vi "Problem 17 - Number letter counts.vi"() -> (3 "Answer = no. of letters used for numbers between 1 and 1,000":i32)   [LabVIEW 2021, in "Project Euler.lvlib"]
uses:
  Project Euler.lvlib
  Utilities/Named Timers/Named Timers.lvlib
panel:
  out "Numbers (Proper English)":string[](array[string])
  out "Total execution time (ms)":u32
  # "Development\nControls or indicators that are useful for development or testing, but which are not outputs of the VI."
  # "Input\nInputs to the VI"
  # "Output\nOutputs of the VI"
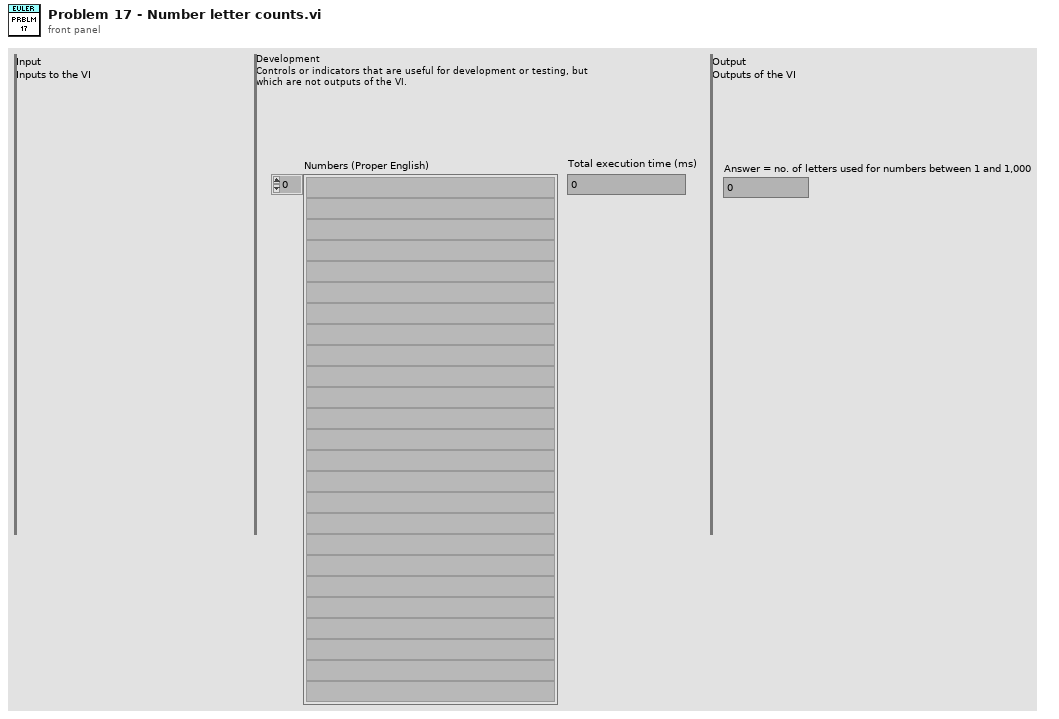
[diagram p1: front panel]
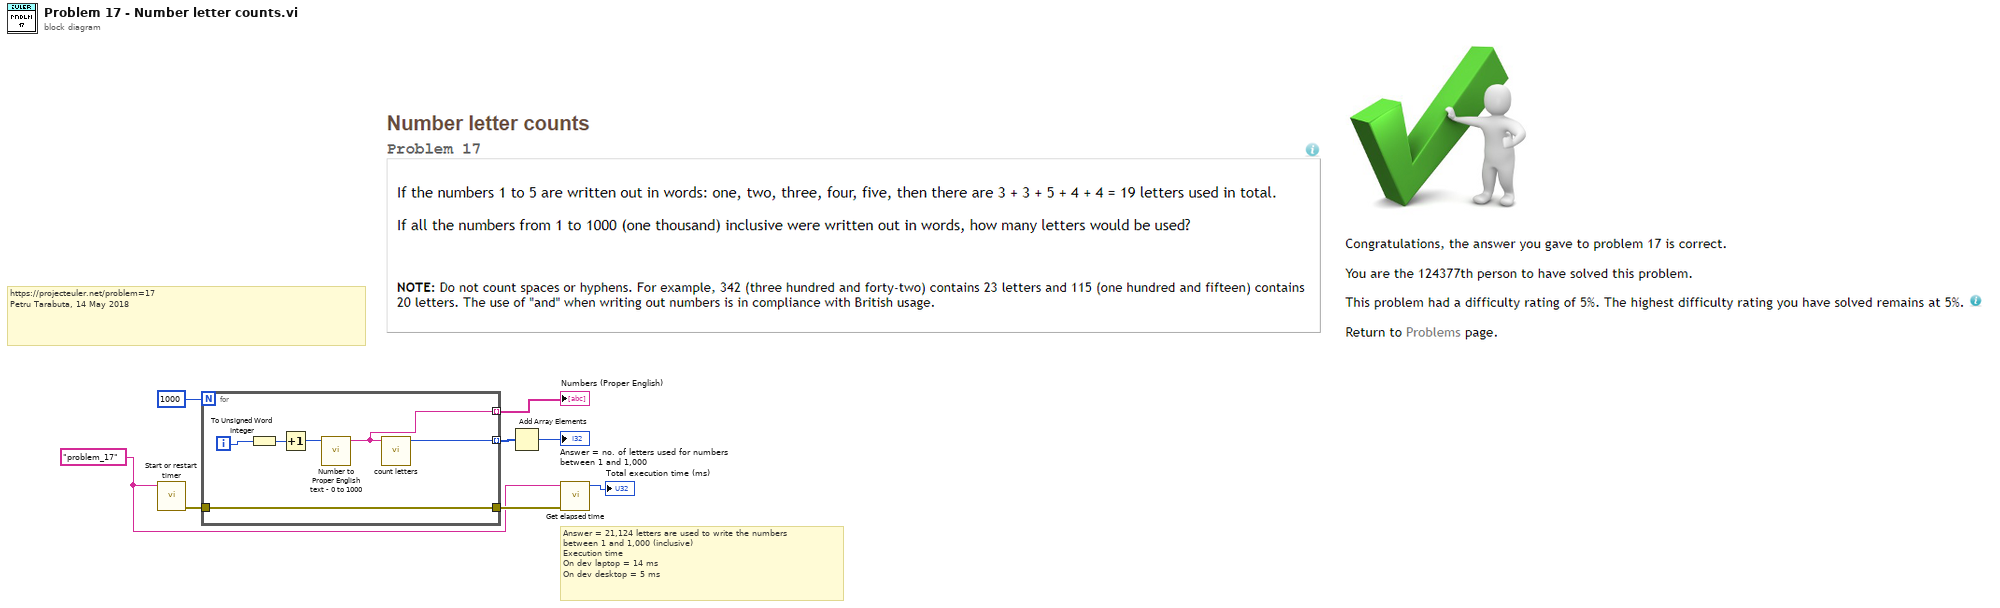
[diagram p0: block diagram]
diagram:
  w1 = "problem_17" ("Timer name")
  # "Answer = 21,124 letters are used to write the numbers between 1 and 1,000 (inclusive)\nExecution time\nOn dev laptop = 14 ms\nOn dev desktop = 5 ms"
  # "https://projecteuler.net/problem=17\nPetru Tarabuta, 14 May 2018"
  n1 = call "Start or restart timer.vi"("Timer name"=w1) -> ("error out"=w3:errorcluster)  [unwired: 10 in]
  n2 = for {
    N: 1000 -> [_]
    tunnel: [w11] -> w6 mode=indexing
    tunnel: [w10] -> w4 mode=indexing
    tunnel: w3 -> [w9]
    tunnel: [w9] -> w2
    i -> [w14]
    n3 = To Unsigned Word Integer(number=w14) -> (unsigned 16bit integer=w12:u16)
    n4 = Increment(x=w12) -> (x+1=w13:u16)
    n5 = call "Number to Proper English text - 0 to 1000.vi"("Positive integer <= 1000"=w13) -> ("Integer written in English"=w11:string)  [unwired: 10 in]
    n6 = call "count letters.vi"("Integer written in English"=w11) -> ("no. of letters"=w10:i32)  [unwired: 10 in]
  }
  "Numbers (Proper English)" <- w6
  n7 = Add Array Elements(numeric array=w4) -> (sum=→"Answer = no. of letters used for numbers between 1 and 1,000":i32)
  n8 = call "Get elapsed time.vi"("error in (no error)"=w2, "Timer name"=w1) -> ("Elapsed time (ms)"=→"Total execution time (ms)":u32)  [unwired: 6 in, 3 out]
